vi "Read Buffer Statistics.vi"(8 "error in (no error)":errorcluster, 11 "VISA resource name":refnum<visa-resource-name>) -> (0 "error out":errorcluster, 1 "Minimum":dbl, 2 "Standard Deviation":dbl, 3 "VISA resource name out":refnum<visa-resource-name>, 4 "Maximum":dbl, 5 "Mean":dbl)   [LabVIEW 2019, in "Keithley 2182.lvlib"]
doc: "Reads data buffer statistics."
uses:
  Keithley 2182.lvlib
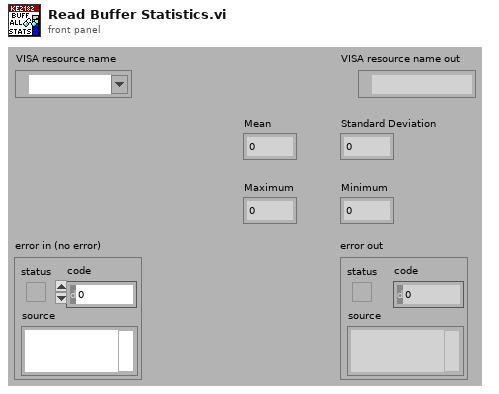
[diagram p1: front panel]
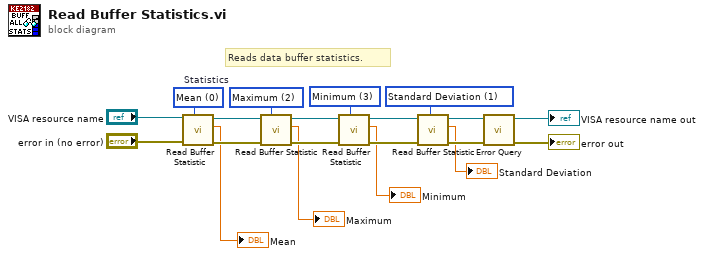
[diagram p0: block diagram]
diagram:
  w17 = u16 1 items=["Mean", "Standard Deviation", "Maximum", "Minimum"] ("Statistic (0: Mean)")
  w18 = u16 3 items=["Mean", "Standard Deviation", "Maximum", "Minimum"] ("Statistic (0: Mean)")
  w19 = u16 2 items=["Mean", "Standard Deviation", "Maximum", "Minimum"] ("Statistic (0: Mean)")
  w20 = u16 0 items=["Mean", "Standard Deviation", "Maximum", "Minimum"]  # Statistics
  # "Reads data buffer statistics."
  n1 = call "Read Buffer Statistic.vi"("Statistic (0: Mean)"=w20, "error in"="error in (no error)", "VISA resource name"="VISA resource name") -> ("error out"=w9:errorcluster, "Statistic Value"=→"Mean":dbl, "VISA resource name out"=w14:refnum<visa-resource-name>)  [unwired: 6 in]
  n2 = call "Read Buffer Statistic.vi"("Statistic (0: Mean)"=w19, "error in"=w9, "VISA resource name"=w14) -> ("error out"=w10:errorcluster, "Statistic Value"=→"Maximum":dbl, "VISA resource name out"=w13:refnum<visa-resource-name>)  [unwired: 6 in]
  n3 = call "Read Buffer Statistic.vi"("Statistic (0: Mean)"=w18, "error in"=w10, "VISA resource name"=w13) -> ("error out"=w11:errorcluster, "Statistic Value"=→"Minimum":dbl, "VISA resource name out"=w12:refnum<visa-resource-name>)  [unwired: 6 in]
  n4 = call "Read Buffer Statistic.vi"("Statistic (0: Mean)"=w17, "error in"=w11, "VISA resource name"=w12) -> ("error out"=w5:errorcluster, "Statistic Value"=→"Standard Deviation":dbl, "VISA resource name out"=w6:refnum<visa-resource-name>)  [unwired: 6 in]
  n5 = call "Error Query.vi"("error in (no error)"=w5, "VISA resource name"=w6) -> ("error out"=→"error out":errorcluster, "VISA resource name out"=→"VISA resource name out":refnum<visa-resource-name>)  [unwired: 6 in, 2 out]
